vi "get action index.vi"(11 "Simple Sequencer TBM runtime in":refnum<class "Simple Sequencer TBM runtime.lvclass">) -> (1 "action index":i32, 3 "Simple Sequencer TBM runtime out":refnum<class "Simple Sequencer TBM runtime.lvclass">)   [LabVIEW 2015, in "Simple Sequencer TBM runtime.lvclass"]
uses:
  Simple Sequencer TBM runtime.lvclass
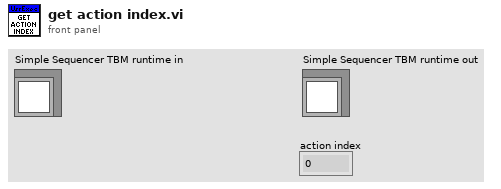
[diagram p1: front panel]
types:
  T1 = typedef "Simple Sequencer TBM runtime.lvclass/meta sequence definition.ctl" = cluster{"sequence length":i32, "sequence pointers":i32[], "continue location":i32}
  T2 = typedef "Simple Sequencer TBM runtime.lvclass/sequence definition.ctl" = cluster{"sequence name":string, "sequence length":i32, "actions with configuration":T3[]}
  T3 = typedef "Simple Sequencer TBM runtime.lvclass/actions with configuration.ctl" = cluster{"action":refnum<class "action.lvclass">, "parameters":T4, "parameters specification":T5[], "results":T4, "results specification":T5[]}
  T4 = typedef "tag bus.lvlib/data table.lvlib/data table.ctl" = cluster{"Double":dbl[], "Single":sgl[], "I64":i64[], "I32":i32[], "I16":i16[], "I8":i8[], "U64":u64[], "U32":u32[], "U16":u16[], "U8":u8[], "Boolean":bool[], "String":string[], "Array of Double":cluster{"DBL Array":dbl[]}[], "Array of Single":cluster{"SGL Array":sgl[]}[], "Array of I64":cluster{"I64 Array":i64[]}[], "Array of I32":cluster{"I32 Array":i32[]}[], "Array of I16":cluster{"I16 Array":i16[]}[], "Array of I8":cluster{"I8 Array":i8[]}[], "Array of U64":cluster{"U64 Array":u64[]}[], "Array of U32":cluster{"U32 Array":u32[]}[], "Array of U16":cluster{"U16 Array":u16[]}[], "Array of U8":cluster{"U8 Array":u8[]}[], "Array of Boolean":cluster{"Boolean Array":bool[]}[], "Array of String":cluster{"String Array":string[]}[]}
  T5 = typedef "tag bus.lvlib/data table.lvlib/transfer specification.ctl" = cluster{"data type":T6, "sink indices":i32[], "source indices":i32[]}
  T6 = typedef "tag bus.lvlib/tag descriptor.lvclass/Data Type.ctl" = enum16{"Double", "Single", "I64", "I32", "I16", "I8", "U64", "U32", "U16", "U8", "Boolean", "String", "Array of Double", "Array of Single", "Array of I64", "Array of I32", "Array of I16", "Array of I8", "Array of U64", "Array of U32", "Array of U16", "Array of U8", "Array of Boolean", "Array of String"}
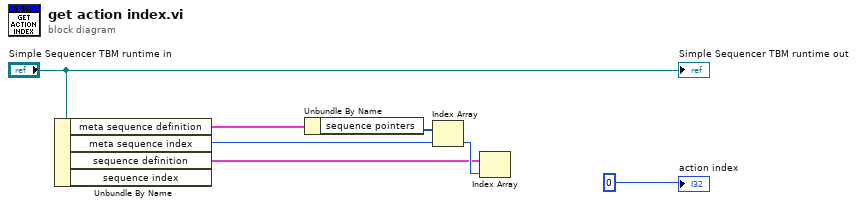
[diagram p0: block diagram]
diagram:
  n1 = Unbundle By Name("Simple Sequencer TBM runtime in") -> ("meta sequence definition"=w5:T1, "meta sequence index"=w4:i32, "sequence definition"=w3:T2[])  [unwired: 1 out]
  n2 = Unbundle By Name(w5) -> ("sequence pointers"=w6:i32[])
  n3 = Index Array(array=w6, index=w4) -> (element=w7:i32)
  n4 = Index Array(array=w3, index=w7) -> ()  [unwired: 1 out]
  "action index" <- 0 ("action index")
  "Simple Sequencer TBM runtime out" <- "Simple Sequencer TBM runtime in"
